vi "Index Motor Value.vi"(1 "Operator X Button":bool) -> (0 "Index Teleop Command":dbl)   [LabVIEW 2019]
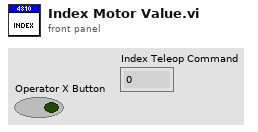
[diagram p1: front panel]
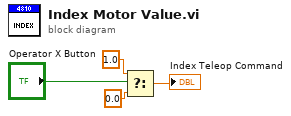
[diagram p0: block diagram]
diagram:
  n1 = Select(t=1.0, s="Operator X Button", f=0.0) -> (s? t:f=→"Index Teleop Command":dbl)
